vi "initializedProgressData.vi"(10 "inputEntry":string[][](array[string])) -> (2 "outputProgressData":string[][](array[string]))   [LabVIEW 2020]
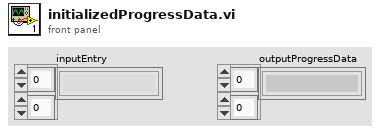
[diagram p1: front panel]
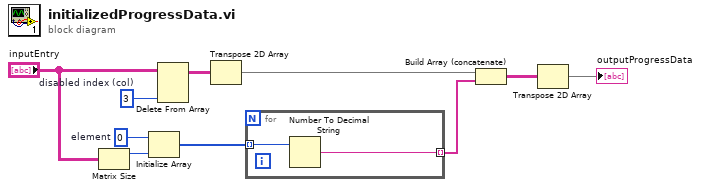
[diagram p0: block diagram]
diagram:
  w6 = 3  # disabled index (col)
  w8 = 0  # element
  n1 = Matrix Size(0:"inputEntry") -> (1:w9:i32)  [unwired: 1 out]
  n2 = Initialize Array "Initialize Array"(w8, w9) -> (w7:i32[])
  n3 = Delete From Array "Delete From Array"(array="inputEntry", index (col)=w6) -> (array with subset deleted=w5:string[][])  [unwired: 2 in, 1 out]
  n4 = Transpose 2D Array(2D array=w5) -> (transposed array=w4:string[][])
  n5 = for {
    tunnel: w7 -> [w12] mode=indexing
    tunnel: [w11] -> w3 mode=indexing
    n6 = Number To Decimal String(number=w12) -> (decimal integer string=w11:string)  [unwired: 1 in]
  }
  n7 = Build Array (concatenate) "Build Array"(w4, w3) -> (w2:string[][])
  n8 = Transpose 2D Array(2D array=w2) -> (transposed array=→"outputProgressData":string[][])
